vi "conteggio_elementi(subVI).vi"(5 "punto 1":i32, 7 "punto 0":i32=1, 8 "error in":errorcluster, 10 "image calibration":path, 11 "Session In":T3="cam0") -> (0 "error out":errorcluster, 2 "Distances":sgl[](array[numeric]) format="%.4f", 3 "number of particle":i32)   [LabVIEW 2020]
uses:
  <vilib>/userDefined/High Color/IMAQdx.ctl
panel:
  in  "Calibration Axis Info":T1={"Origin Pixel"={"X"=0.0, "Y"=0.0}, "Angle Relative to Horizontal (deg)"=0.0, "Axis Reference"=1} {"Axis Reference" items=["Direct", "Indirect"]}
  in  "?":bool
  out "Image":T2(plugin-control)
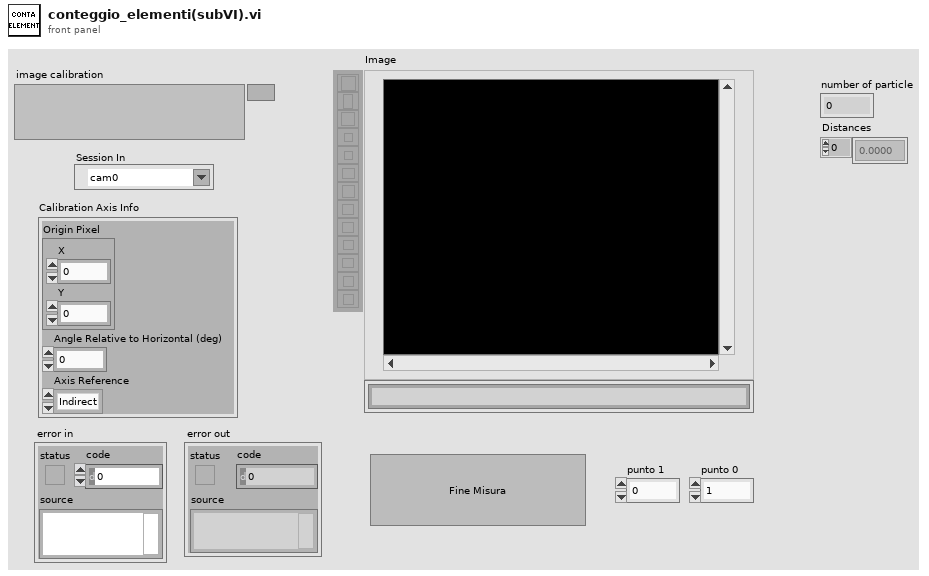
[diagram p1: front panel]
types:
  T1 = cluster{"Origin Pixel":cluster{"X":sgl, "Y":sgl}, "Angle Relative to Horizontal (deg)":sgl, "Axis Reference":u32}
  T2 = typedef "IMAQ Image.ctl" = refnum<image>
  T3 = typedef "IMAQdx.ctl" = refnum<k21>
  T4 = typedef "Image Type" = u32
  T5 = cluster{"Area":dbl, "Number of Holes":dbl, "Bounding Rect":cluster{"Left":dbl, "Top":dbl, "Right":dbl, "Bottom":dbl}, "Center of Mass":cluster{"X":dbl, "Y":dbl}, "Orientation":dbl, "Dimensions":cluster{"Width":dbl, "Height":dbl}}[]
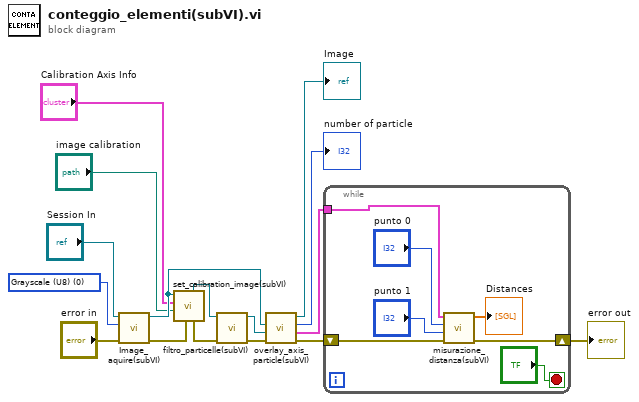
[diagram p0: block diagram]
diagram:
  w14 = T4 0 items=["Grayscale (U8)", "Grayscale (I16)", "Grayscale (SGL)", "Complex (CSG)", "RGB (U32)", "HSL (U32)", "RGB (U64)", "Grayscale (U16)"] ("Image Type")
  n1 = call "Image_aquire(subVI).vi"("error in"="error in", "Image Type"=w14, "Session In"="Session In") -> ("error out"=w7:errorcluster, "Grey scale image"=w5:T2)  [unwired: 6 in, 1 out]
  n2 = call "set_calibration_image(subVI).vi"("error in (no error)"=w7, "File Path"="image calibration", "Calibration Axis Info"="Calibration Axis Info", "Image Dst"=w5) -> ("error out"=w6:errorcluster, "Image Out"=w4:T2)  [unwired: 5 in, 1 out]
  n3 = call "filtro_particelle(subVI).vi"("error in (no error)"=w6, "Image Src"=w4) -> ("error out"=w1:errorcluster, "Image"=w8:T2)  [unwired: 8 in]
  n4 = call "overlay_axis_particle(subVI).vi"("error in (no error)"=w1, "filtred & calibrated image"=w8, "view image"=w5) -> ("error out"=w11:errorcluster, "Particle Reports (Real-World)"=w9:T5, "number of particle"=→"number of particle":i32, "Image Out"=→"Image":T2)  [unwired: 5 in]
  n5 = while {
    tunnel: w9 -> [w19]
    shift-right: [w21] -> w10
    shift-left: w11 -> [w22]
    stop <- "?" stop-if-true
    n6 = call "misurazione_distanza(subVI).vi"("error in (no error)"=w22, "punto 1"="punto 1", "punto 0"="punto 0", "particle reports (real-world)"=w19) -> ("error out"=w21:errorcluster, "Distances"=→"Distances":sgl[])  [unwired: 6 in]
  }
  "error out" <- w10
